vi "PID.vi"() -> ()   [LabVIEW 2013]
uses:
  <vilib>/Platform/TimedLoop/XDataNode/timing_clust.ctl
  <vilib>/Platform/TimedLoop/XDataNode/nitl_modes.ctl
  <vilib>/Platform/TimedLoop/XDataNode/wakeup.ctl
  <vilib>/platform/TimedLoop/XDataNode/XDataNode.xnode
  <vilib>/Platform/TimedLoop/XDataNode/XDNodeRunTimeDep.lvlib
  <vilib>/LabVIEW Interface for Arduino/LabVIEW Interface for Arduino.lvlib
panel:
  out "Salida PWM":dbl
  out "Temp":dbl
  out "Grafica":cluster{"Referencia":dbl, dbl, "u":dbl}(graph)
  out "Temperatura":dbl(slide) scale=0.0..50.0
  in  "?":bool
  in  "Puerto Salida PWM":u8=3
  in  "Puerto entrada analogica":u8
  in  "KI":dbl
  in  "KD":dbl
  in  "KP":dbl
  in  "Referencia":dbl
  # "CONTROL PID"
  # "INSTITUTO TECNOLÓGICO SUPERIOR DE CIUDAD HIDALGO\n\n                            MATERIA: CONTROL DE PROCESOS\n\n                          CARRERA: ING. MECATRÓNICA\n\n                                         SEMESTRE: 9\n\n                                         GRUPO: 359G\n                                        \n                      JOSE NOEL DOMINGUEZ MIRALRIO\n                 LEONARDO GARIBALDI GARFIAS PANIAGUA\n                               ERNESTO MARTINEZ AVILA\n                      CERSAR FRANCISCO FRANCISCO \n                            ERICK VILLEGAS GONZALES\n                                JUAN MANUEL MALDONADO CRUZ\n                                         EDGAR AGUILAR RODEA\n                              LEONARDO GARIBALDI GARFIAS PANIAGUA"
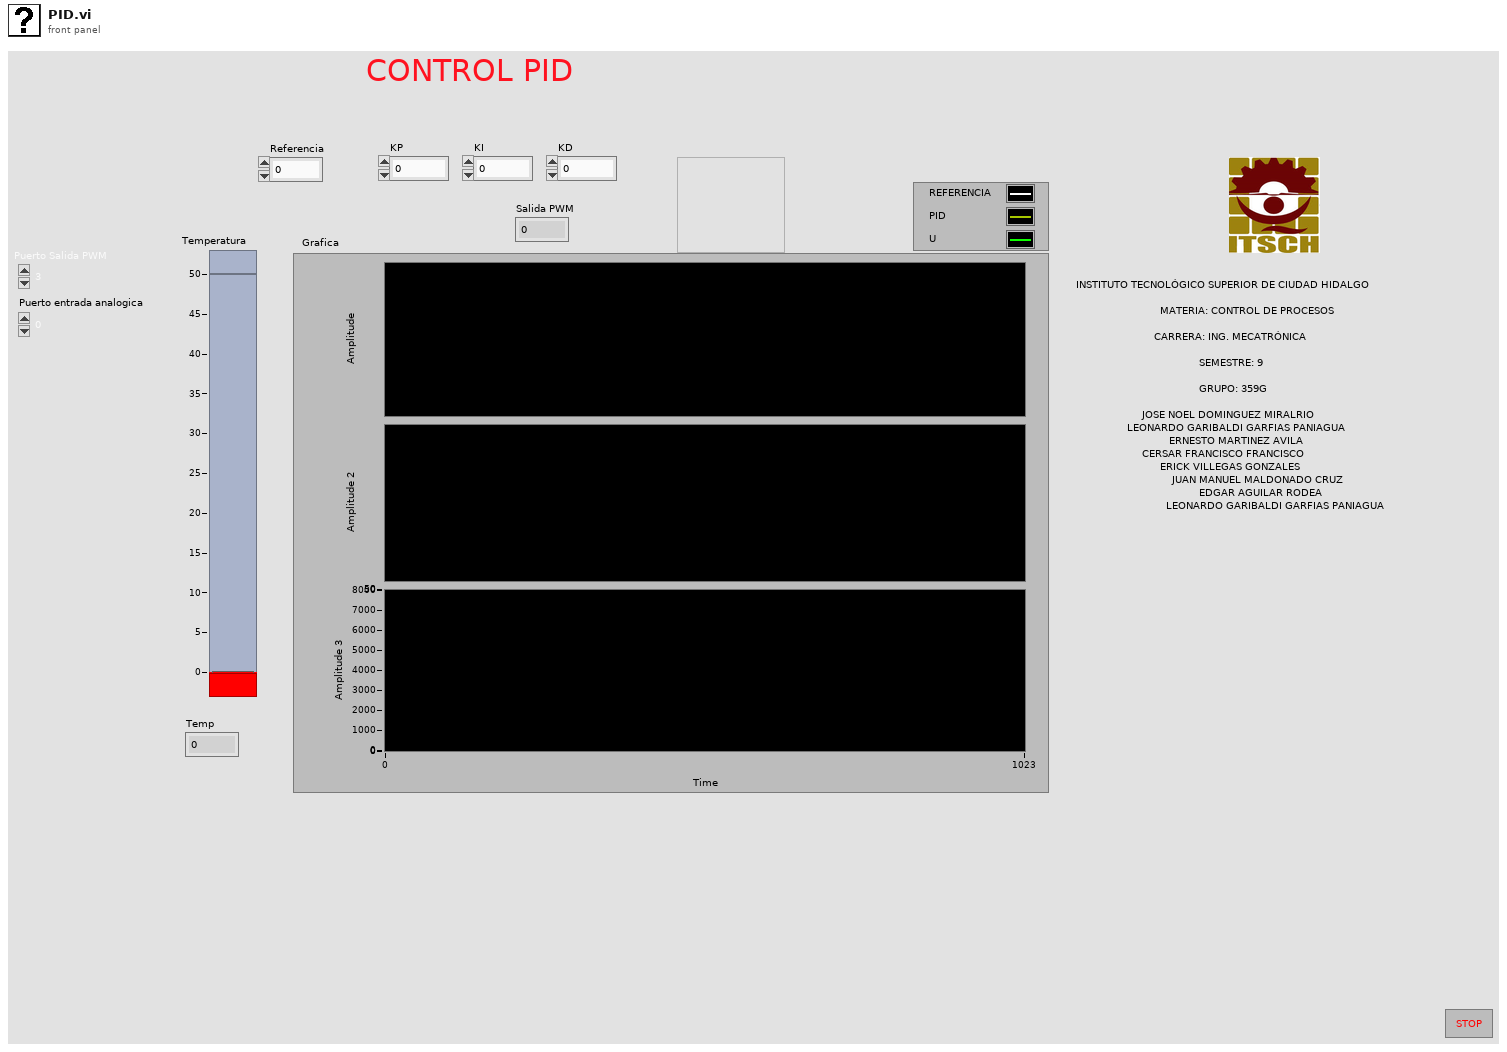
[diagram p1: front panel]
types:
  T1 = typedef "XDNodeRunTimeDep.lvlib/timing_clust.ctl" = cluster{"Expected End [f-1]":u64, "Actual End [f-1]":u64, "Finished Late? [f-1]":bool, "Expected End [i-1]":u64, "Actual End [i-1]":u64, "Finished Late? [i-1]":bool, "Expected Start [i]":u64, "Actual Start [i]":u64, "Expected Start [f]":u64, "Actual Start [f]":u64, "Source Name":string, "Structure Name":string, "Period":i64, "Deadline":i64, "Offset":i64, "Start":i64, "Priority":i32, "Timeout":i32, "Mode":T2, "Wakeup Reason":T3, "Error":errorcluster, "Source Type":string, "Secondary Source Type":string, "Global End Time":u64, "Global Start Time":u64, "Frame Duration":u64, "Iteration Duration":u64, "Assigned CPU":i32, "I/O Scan Engine Mode":u32}
  T2 = typedef "XDNodeRunTimeDep.lvlib/nitl_modes.ctl" = enum32{"No Change", "Process missed periods, maintain original phase", "Discard missed periods, maintain original phase", "Process missed periods, ignore original phase", "Discard missed periods, ignore original phase"}
  T3 = typedef "XDNodeRunTimeDep.lvlib/wakeup.ctl" = enum32{"Normal", "Aborted", "Asynchronous wakeup", "Timing source error", "Timed loop error", "Timeout"}
  T4 = typedef "LabVIEW Interface for Arduino.lvlib/Arduino Resource.ctl" = cluster{"VISA resource":refnum<visa-resource-name>, "Board Type":T5, "Connection Type":enum8{"USB / Serial"}, "Bytes Per Packet (15)":u8}
  T5 = typedef "LabVIEW Interface for Arduino.lvlib/Board Type.ctl" = enum16{"Uno", "Dimuelanove w/Atmega 328", "Mega 2560"}
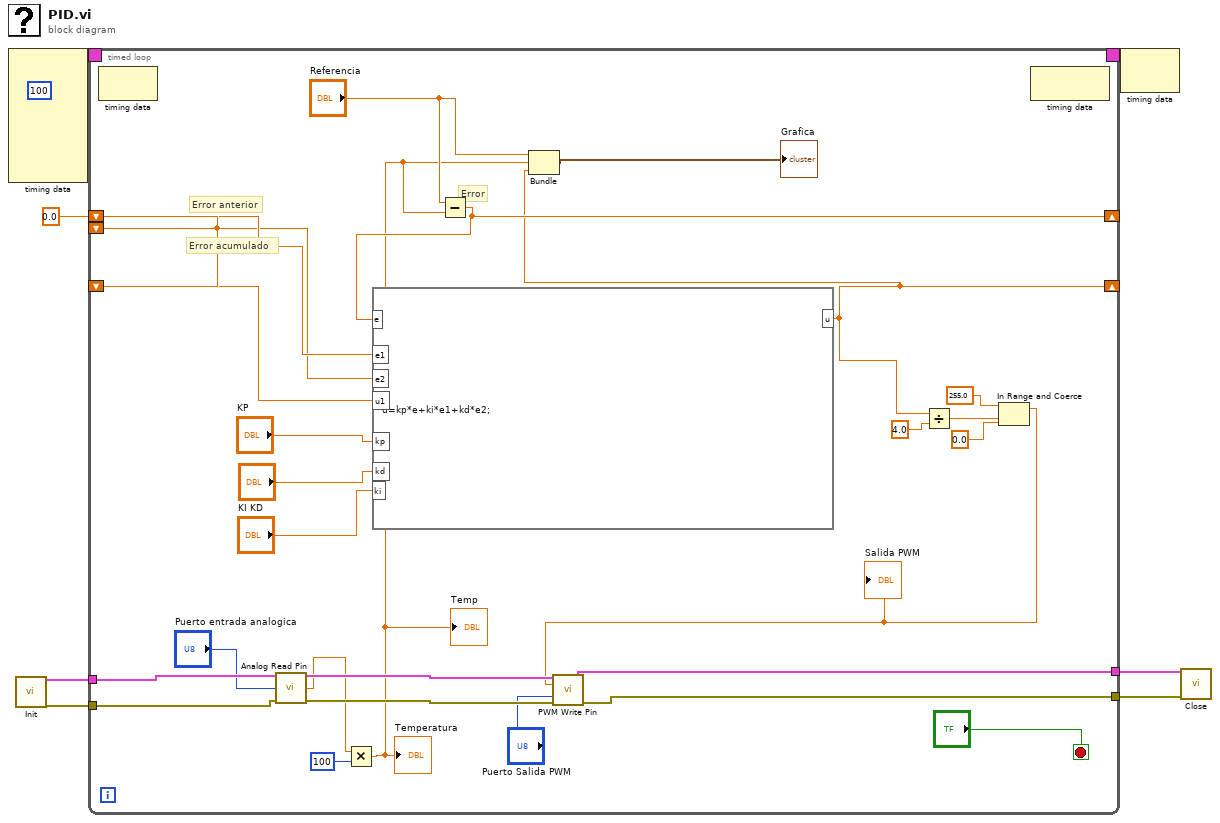
[diagram p0: block diagram]
diagram:
  w6 = 0.0
  n1 = node-c288(i64 100 ("Period")) -> (w8:T1)  [unwired: 6 in]
  n2 = call <vilib>:"Init.vi"() -> ("Arduino Resource"=w5:T4, "error out"=w4:errorcluster)  [unwired: 18 in]
  n3 = timed-loop {
    timing: w8 -> [_]
    timing-out: [_] -> w7
    shift-right: [w33] -> _
    shift-left: w6 -> [w32]
    shift-left: w6 -> [w31]
    shift-right: [w9] -> _
    shift-left: w6 -> [w34]
    tunnel: w5 -> [w27]
    tunnel: w4 -> [w26]
    tunnel: [w24] -> w3
    tunnel: [w22] -> w2
    stop <- "?" stop-if-true
    # "Error acumulado"
    # "Error anterior"
    # "Error"
    n4 = node-c288() -> ()  [unwired: 1 in, 1 out]
    n5 = call <vilib>:"Analog Read Pin.vi"("Arduino Resource"=w27, "Analog Input Pin (0)"="Puerto entrada analogica", "error in"=w26) -> ("Arduino Resource"=w25:T4, "Voltage"=w14:dbl, "error out"=w23:errorcluster)  [unwired: 10 in]
    n6 = Multiply(x=w14, y=u8 100) -> (x*y=w12:dbl)
    "Temperatura" <- w12
    "Temp" <- w12
    n7 = Subtract(x="Referencia", y=w12) -> (x-y=w33:dbl)
    n8 = formula code="u=kp*e+ki*e1+kd*e2;"("e"=w33, "e1"=w32, "e2"=w31, "u1"=w34, "kp"="KP", "kd"="KD", "ki"="KI") -> ("u"=w9:dbl)
    n9 = Bundle("Referencia"="Referencia", w12, "u"=w9) -> (→"Grafica":cluster{"Referencia":dbl, dbl, "u":dbl})  [unwired: 1 in]
    n10 = Divide(x=w9, y=4.0) -> (x/y=w13:dbl)
    n11 = In Range and Coerce(upper limit=255.0, x=w13, lower limit=0.0) -> (coerced(x)=w11:dbl)  [unwired: 1 out]
    "Salida PWM" <- w11
    n12 = call <vilib>:"PWM Write Pin.vi"("Arduino Resource"=w25, "Duty Cycle (0 - 255)"=w11, "PWM Pin (3)"="Puerto Salida PWM", "error in"=w23) -> ("Arduino Resource"=w24:T4, "error out"=w22:errorcluster)  [unwired: 10 in]
    n13 = node-c288() -> ()  [unwired: 1 in, 1 out]
  }
  n14 = node-c288(w7) -> ()  [unwired: 1 out]
  n15 = call <vilib>:"Close.vi"("Arduino Resource"=w3, "error in"=w2) -> ()  [unwired: 13 in, 1 out]
